vi "sub.vi"(4 "Physical Channel":tag="PXIe_NI6341/ai0:1", 5 "Number of Samples in":i32=100, 6 "Max Voltage":dbl=5.0, 7 "Sample Rate":dbl=1000.0, 9 "Sample Clock Source":tag="OnboardClock", 10 "Min Voltage":dbl=-5.0, 11 "Terminal Configuration":i32(ring)=10083 items=["default"=-1, "RSE"=10083, "NRSE"=10078, "Differential"=10106, "Pseudodifferential"=12529]) -> (0 "error out":errorcluster, 1 "Actual Sample Rate":dbl=1000.0 format="%0.2f", 2 "Number of Samples out":i32=100, 3 "Refnum out":refnum<k21>)   [LabVIEW 2018]
uses:
  <vilib>/DAQmx/create/channels.llb/DAQmx Create Channel (AI-Voltage-Basic).vi
  <vilib>/DAQmx/configure/timing.llb/DAQmx Timing (Sample Clock).vi
  <resource>/objmgr/daqmx.rc
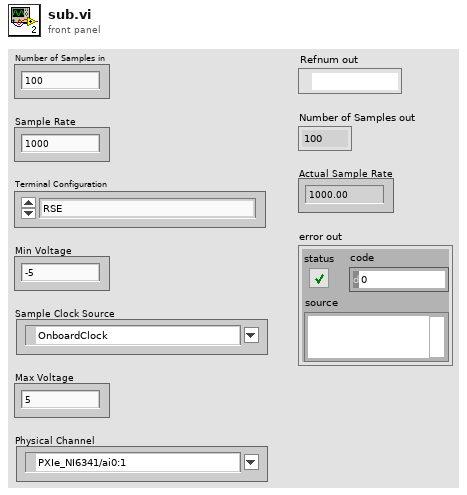
[diagram p1: front panel]
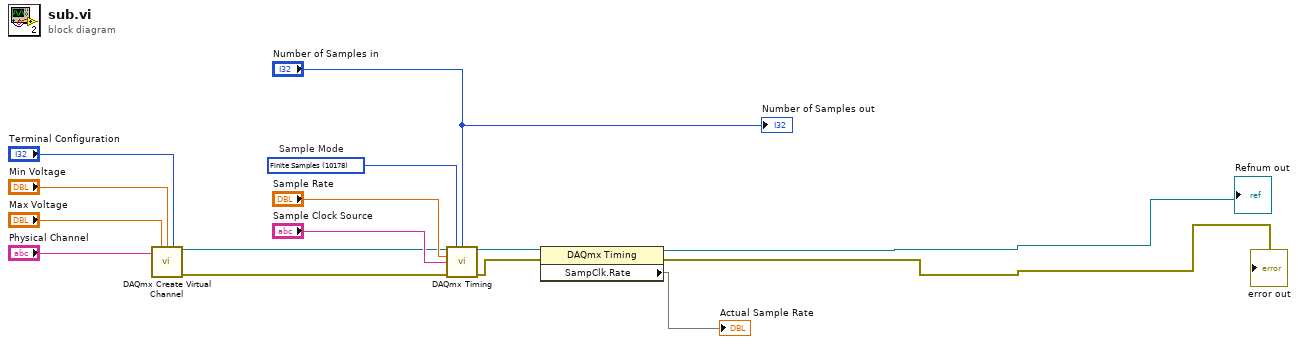
[diagram p0: block diagram]
diagram:
  w5 = 10178 items=["Finite Samples"=10178, "Continuous Samples"=10123, "Hardware Timed Single Point"=12522]  # Sample Mode
  n1 = call-poly <vilib>:"DAQmx Create Virtual Channel.vi"("maximum value"="Max Voltage", "minimum value"="Min Voltage", "input terminal configuration"="Terminal Configuration", "physical channels"="Physical Channel") -> ("task out"=w7:refnum<k21>, "error out"=w6:errorcluster)  [unwired: 10 in]
  n2 = call-poly <vilib>:"DAQmx Timing.vi"("task/channels in"=w7, "sample mode"=w5, "samples per channel"="Number of Samples in", "rate"="Sample Rate", "source"="Sample Clock Source", "error in"=w6) -> ("task out"=w3:refnum<k21>, "error out"=w4:errorcluster)  [unwired: 8 in]
  n3 = property class="DAQmx Timing"(reference=w3, error in=w4) -> (reference out=→"Refnum out":refnum<k21>, error out=→"error out":errorcluster, "SampClk.Rate"=→"Actual Sample Rate")
  "Number of Samples out" <- "Number of Samples in"
